vi "HexUtility.vi"() -> ()   [LabVIEW 2021]
panel:
  out "VX Most Significant Bit":u8 format="%08b"
  out "VX shifted left 1":u8 format="%08b"
  out "Exclusive XOR":u8 format="%08b"
  out "Not Exclusive XOR":u8 format="%08b"
  in  "VY":u8 format="%08b"
  out "LSB of VX":u8 format="%08b"
  out "VX shifted right 1":u8 format="%08b"
  out "VX + I":u16 format="%04x"
  in  "VX":u8 format="%08b"
  in  "I":u16 format="%04x"
  out "Binary XOR Result":u8 format="%08b"
  out "AND 000F":u16 format="%04x"
  out "VX Decimal":u8 format="%02d"
  out "VX":u8 format="%02x"
  out "NN":u8 format="%02x"
  out "0NNN":bool
  out "00EE":bool
  out "00E0":bool
  out "AND F000 after Case Selector":u16 format="%04x"
  out "AND F000? Binary":u16 format="%0b"
  in  "Hex 2":u8 format="%02x"
  out "Binary AND Result":u8 format="%08b"
  in  "Hex 1":u8 format="%02x"
  out "AND F000?":u16 format="%04x"
  out "Typecast Memory at PC":u16 format="%04x"
  out "Memory at PC+1":u8 format="%02x"
  out "Memory At PC+1 Swapped":u16 format="%04x"
  out "Memory At PC":u8 format="%02x"
  out "Opcode Generated":u16 format="%04x"
  in  "PC":u16=512 format="%x"
  in  "Memory":u8[](array[numeric]) format="%02x"
  out "Decimal":u16 format="%0d"
  in  "Hex":u16 format="%04x"
  # "Each position = 1 byte"
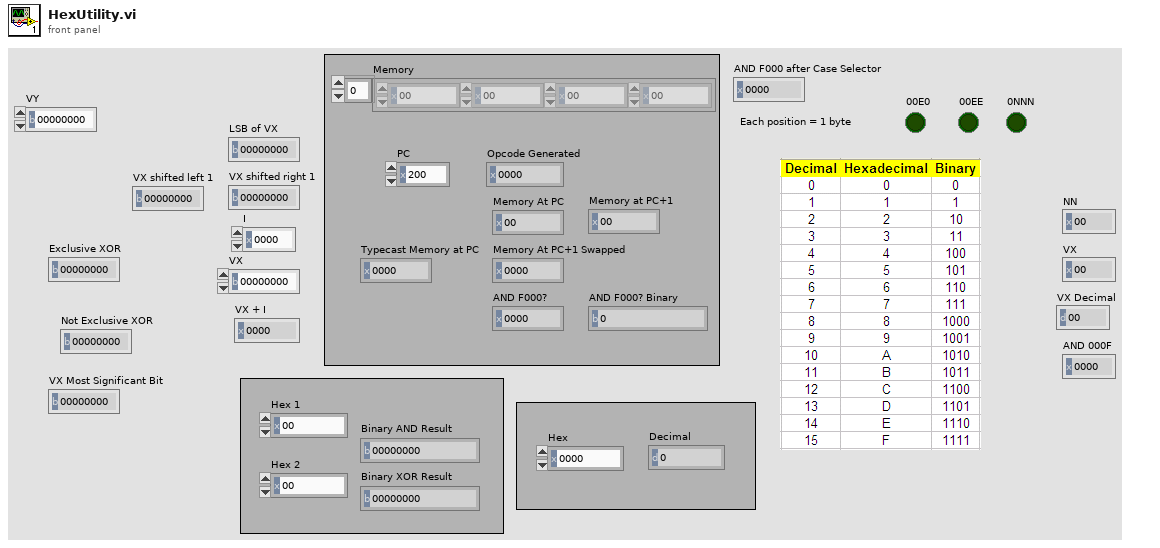
[diagram p1: front panel]
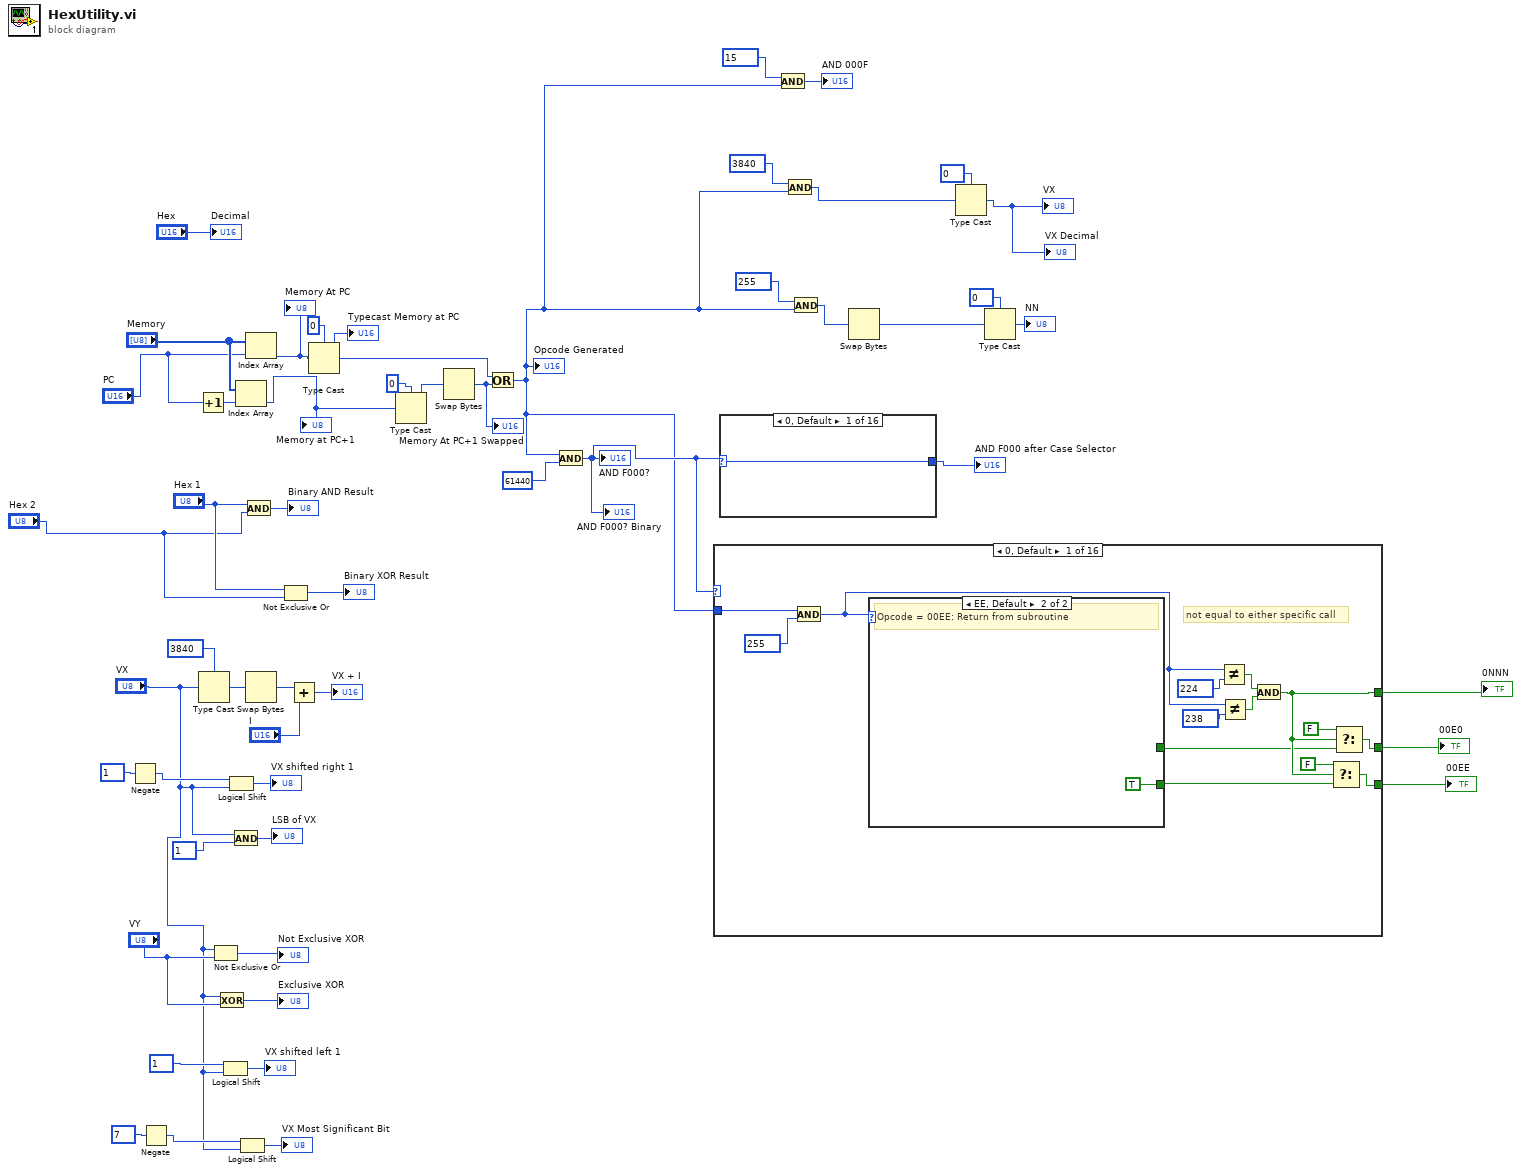
[diagram p0: block diagram]
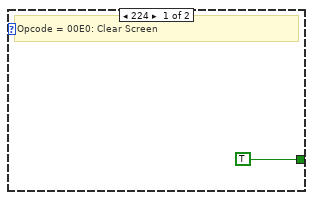
[diagram p2: hidden frame]
diagram:
  n1 = Negate(x=i8 1 ("y")) -> (-x=w13:i8)
  n2 = Negate(x=i8 7 ("y")) -> (-x=w3:i8)
  n3 = Increment(x="PC") -> (x+1=w51:u16)
  n4 = Type Cast(type=u16 3840 ("y"), x="VX") -> (*(type *) &x=w19:u16)
  n5 = Not Exclusive Or(1:"VY", 2:"VX") -> (0:→"Not Exclusive XOR":u8)
  n6 = Exclusive Or(1:"VY", 2:"VX") -> (0:→"Exclusive XOR":u8)
  n7 = Logical Shift(y=i8 1, x="VX") -> (x << y=→"VX shifted left 1":u8)
  n8 = Logical Shift(y=w13, x="VX") -> (x << y=→"VX shifted right 1":u8)
  n9 = And(x="VX", y=u8 1) -> (x .and. y?=→"LSB of VX":u8)
  n10 = Index Array(array="Memory", index=w51) -> (element=w47:u8)
  "Memory at PC+1" <- w47
  n11 = Logical Shift(y=w3, x="VX") -> (x << y=→"VX Most Significant Bit":u8)
  n12 = And(x="Hex 1", y="Hex 2") -> (x .and. y?=→"Binary AND Result":u8)
  n13 = Index Array(array="Memory", index="PC") -> (element=w45:u8)
  "Memory At PC" <- w45
  n14 = Swap Bytes(anything=w19) -> (byte swapped=w15:u16)
  n15 = Not Exclusive Or(1:"Hex 2", 2:"Hex 1") -> (0:→"Binary XOR Result":u8)
  n16 = Add(x=w15, y="I") -> (x+y=→"VX + I":u16)
  n17 = Type Cast(type=u16 0, x=w45) -> (*(type *) &x=w43:u16)
  "Typecast Memory at PC" <- w43
  n18 = Type Cast(type=u16 0, x=w47) -> (*(type *) &x=w46:u16)
  n19 = Swap Bytes(anything=w46) -> (byte swapped=w40:u16)
  "Memory At PC+1 Swapped" <- w40
  n20 = Or(x=w43, y=w40) -> (x .or. y?=w24:u16)
  "Opcode Generated" <- w24
  n21 = And(x=w24, y=u16 61440) -> (x .and. y?=w38:u16)
  "AND F000?" <- w38
  "AND F000? Binary" <- w38
  n22 = case shown="0, Default" w38 {
    tunnel: w24 -> [w54 _ _ _ _ _ _ _ _ _ _ _ _ _ _ _]
    tunnel: [w56 _ _ _ _ _ _ _ _ _ _ _ _ _ _ _] -> w37
    tunnel: [w58 _ _ _ _ _ _ _ _ _ _ _ _ _ _ _] -> w36
    tunnel: [w57 _ _ _ _ _ _ _ _ _ _ _ _ _ _ _] -> w35
    frame 0, Default {
      # "not equal to either specific call"
      n23 = And(x=w54, y=u16 255) -> (x .and. y?=w53:u16)
      n24 = case shown="EE, Default" w53 {
        tunnel: [_ TRUE ("00EE")] -> w61
        tunnel: [TRUE ("00E0") _] -> w55
        frame 224 {
          # "Opcode = 00E0: Clear Screen"
        }
        frame 238, Default {
          # "Opcode = 00EE: Return from subroutine"
        }
      }
      n25 = Not Equal?(x=w53, y=u16 224) -> (x != y?=w64:bool)
      n26 = Not Equal?(x=w53, y=u16 238) -> (x != y?=w65:bool)
      n27 = And(x=w64, y=w65) -> (x .and. y?=w56:bool)
      n28 = Select(t=FALSE, s=w56, f=w61) -> (s? t:f=w58:bool)
      n29 = Select(t=FALSE, s=w56, f=w55) -> (s? t:f=w57:bool)
    }
    frame 4096 {
    }
    frame 8192 {
    }
    frame 12288 {
    }
    frame 16384 {
    }
    frame 20480 {
    }
    frame 24576 {
    }
    frame 28672 {
    }
    frame 32768 {
    }
    frame 36864 {
    }
    frame 40960 {
    }
    frame 45056 {
    }
    frame 49152 {
    }
    frame 53248 {
    }
    frame 57344 {
    }
    frame 61440 {
    }
  }
  "0NNN" <- w37
  "00EE" <- w36
  "00E0" <- w35
  n30 = case shown="0, Default" w38 {
    selector: w38 -> [w69 w70 w71 w72 w73 w74 w75 w76 w77 w78 w79 w80 w81 w82 w83 w84]
    tunnel: [w69 w70 w71 w72 w73 w74 w75 w76 w77 w78 w79 w80 w81 w82 w83 w84] -> w39
    frame 0, Default {
    }
    frame 4096 {
    }
    frame 8192 {
    }
    frame 12288 {
    }
    frame 16384 {
    }
    frame 20480 {
    }
    frame 24576 {
    }
    frame 28672 {
    }
    frame 32768 {
    }
    frame 36864 {
    }
    frame 40960 {
    }
    frame 45056 {
    }
    frame 49152 {
    }
    frame 53248 {
    }
    frame 57344 {
    }
    frame 61440 {
    }
  }
  "AND F000 after Case Selector" <- w39
  n31 = And(x=u16 15 ("y"), y=w24) -> (x .and. y?=→"AND 000F":u16)
  n32 = And(x=u16 3840 ("y"), y=w24) -> (x .and. y?=w28:u16)
  n33 = And(x=u16 255 ("y"), y=w24) -> (x .and. y?=w33:u16)
  n34 = Swap Bytes(anything=w33) -> (byte swapped=w30:u16)
  n35 = Type Cast(type=u8 0, x=w28) -> (*(type *) &x=→"VX" →"VX Decimal":u8)
  n36 = Type Cast(type=u8 0, x=w30) -> (*(type *) &x=→"NN":u8)
  "Decimal" <- "Hex"
